vi "Gaussian_fit_SubV).vi"(0 "Fit model":refnum<vi>, 1 "sub array buffer":i16, 2 "initial parameters":dbl[](array[numeric]), 3 "Cluster":T1, 4 "Image Index":i32, 6 "Fit position":cluster{"X":i32, "Y":i32}, 7 "Image Array":u16[][](array[numeric]), 9 "Array 3":dbl[][](array[numeric])) -> (8 "Value 3":cluster{"X":i32, "Y":i32}, 10 "number of function calls":i32, 11 "Array":u16[][](array[numeric]), 12 "best nonlinear fit":dbl[][](array[numeric]), 13 "best fit parameters":dbl[](array[numeric]), 14 "Numeric 4":dbl, 15 "Numeric 3":dbl, 16 "Numeric out":dbl, 17 "Array 2":dbl[][](array[numeric]), 18 "residue":dbl)   [LabVIEW 2012]
uses:
  <vilib>/gmath/NumericalOptimization/Nonlinear Curve Fit LM.vi
  <vilib>/gmath/NI_Gmath.lvlib
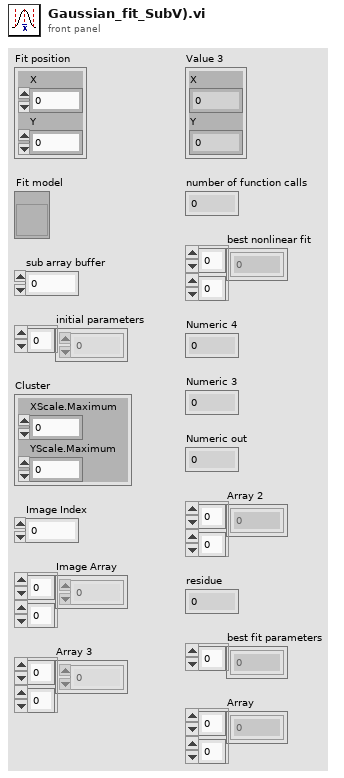
[diagram p1: front panel]
types:
  T1 = cluster{"XScale.Maximum":dbl, "YScale.Maximum":dbl}
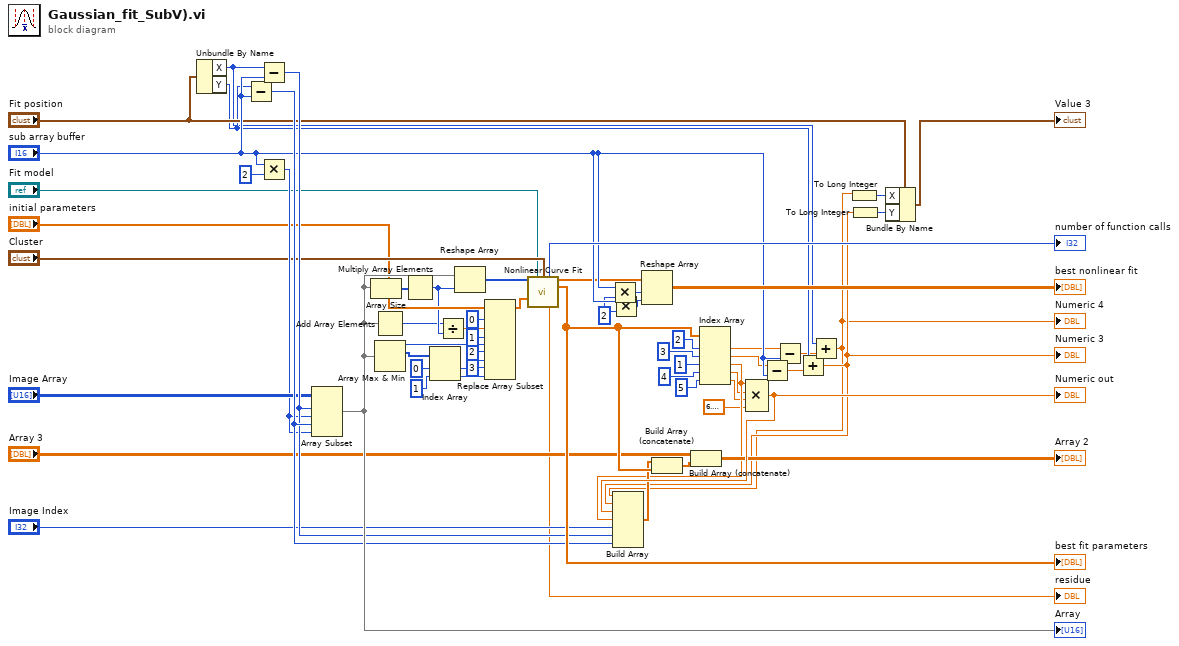
[diagram p0: block diagram]
diagram:
  w35 = i16 2 ("y")
  n1 = Unbundle By Name("Fit position") -> ("X"=w25:i32, "Y"=w26:i32)
  n2 = Subtract(x=w26, y="sub array buffer") -> (x-y=w56:i32)
  n3 = Subtract(x=w25, y="sub array buffer") -> (x-y=w55:i32)
  n4 = Multiply(x="sub array buffer", y=i16 2) -> (x*y=w43:i16)
  n5 = Array Subset(array="Image Array", index (row)=w55, length (row)=w43, index (col)=w56, length (col)=w43) -> (w61:u16[][])
  "Array" <- w61
  n6 = Array Size(array=w61) -> (size(s)=w1:i32[])
  n7 = Add Array Elements(numeric array=w61) -> (sum=w12:u16)
  n8 = Array Max & Min(array=w61) -> (max value=w11:u16, max index (indices)=w3:i32[])  [unwired: 2 out]
  n9 = Multiply Array Elements(1:w1) -> (0:w16:i32)
  n10 = Index Array(array=w3, index #1=0 ("index"), index #2=1 ("index")) -> (element #1=w10:i32, element #2=w9:i32)
  n11 = Divide(x=w12, y=w16) -> (x/y=w14:dbl)
  n12 = Reshape Array(w61, w16) -> (w2:u16[])
  n13 = Replace Array Subset(array="initial parameters", new element #1=w14, index #1=0 ("index"), new element #2=w11, index #2=1 ("index"), new element #3=w10, index #3=2 ("index"), new element #4=w9, index #4=3 ("index")) -> (w8:dbl[])
  n14 = call-poly <vilib>:"Nonlinear Curve Fit.vi"("Y"=w2, "f(x,a)"="Fit model", "data"="Cluster", "initial parameters"=w8) -> ("number of function calls"=→"number of function calls":i32, "best nonlinear fit"=w31:dbl[], "best fit parameters"=w60:dbl[], "residue"=→"residue":dbl)  [unwired: 6 in, 2 out]
  "best fit parameters" <- w60
  n15 = Multiply(x="sub array buffer", y=w35) -> (x*y=w34:i16)
  n16 = Multiply(x="sub array buffer", y=w35) -> (x*y=w33:i16)
  n17 = Reshape Array(w31, w34, w33) -> (→"best nonlinear fit":dbl[][])
  n18 = Index Array(array=w60, index #1=2 ("index"), index #2=3 ("index"), index #3=1 ("index"), index #4=4 ("index"), index #5=5 ("index")) -> (element #1=w22:dbl, element #2=w21:dbl, element #3=w49:dbl, element #4=w41:dbl, element #5=w42:dbl)
  n19 = Compound Arithmetic op=MULTIPLY(w49, w41, w42, 6.283185307179586) -> (w59:dbl)
  "Numeric out" <- w59
  n20 = Subtract(x=w21, y="sub array buffer") -> (x-y=w24:dbl)
  n21 = Subtract(x=w22, y="sub array buffer") -> (x-y=w23:dbl)
  n22 = Add(x=w26, y=w24) -> (x+y=w48:dbl)
  "Numeric 3" <- w48
  n23 = Add(x=w25, y=w23) -> (x+y=w47:dbl)
  "Numeric 4" <- w47
  n24 = Build Array(w47, w48, w59, w49, "Image Index", w55, w56) -> (w53:dbl[])
  n25 = Build Array (concatenate)(w53, w60) -> (w54:dbl[])
  n26 = Build Array (concatenate)("Array 3", w54) -> (→"Array 2":dbl[][])
  n27 = To Long Integer(number=w47) -> (32bit integer=w28:i32)
  n28 = To Long Integer(number=w48) -> (32bit integer=w29:i32)
  n29 = Bundle By Name(cluster="Fit position", "X"=w28, "Y"=w29) -> (→"Value 3":cluster{"X":i32, "Y":i32})
